vi "数据索引起始时间填补空白.vi"(8 "error in (no error)":errorcluster caption="错误输入（无错误）") -> (0 "error out":errorcluster caption="错误输出")   [LabVIEW 2016, in "数据传输系统.lvlib"]
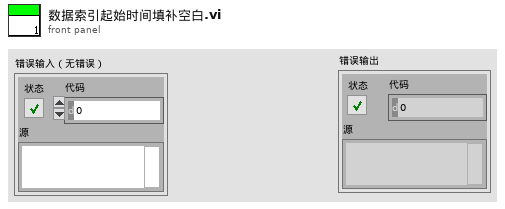
[diagram p1: front panel]
types:
  T1 = typedef "LVDateTimeRec.ctl" = cluster{"秒数的小数部分":dbl, "秒":i32, "分":i32, "时":i32, "日":i32, "月":i32, "年":i32, "天数（周）":i32, "天数（年）":i32, "DST":i32}
  T2 = cluster{"氨氮仪器参数索引起始时间":string, "总磷仪器参数索引起始时间":string, "总氮仪器参数索引起始时间":string, "CODMn仪器参数索引起始时间":string, "CODCr仪器参数索引起始时间":string, "DO仪器参数索引起始时间":string, "PH仪器参数索引起始时间":string, "比电导率仪器参数索引起始时间":string, "水温仪器参数索引起始时间":string, "浊度仪器参数索引起始时间":string, "叶绿素a仪器参数索引起始时间":string, "藻密度仪器参数索引起始时间":string, "ORP仪器参数索引起始时间":string}
  T3 = cluster{"氨氮标样核查索引起始时间":string, "总磷标样核查索引起始时间":string, "总氮标样核查索引起始时间":string, "CODMn标样核查索引起始时间":string, "CODCr标样核查索引起始时间":string, "DO标样核查索引起始时间":string, "PH标样核查索引起始时间":string, "比电导率标样核查索引起始时间":string, "水温标样核查索引起始时间":string, "浊度标样核查索引起始时间":string, "叶绿素a标样核查索引起始时间":string, "藻密度标样核查索引起始时间":string, "亚硝酸盐标样核查索引起始时间":string, "硫化物标样核查索引起始时间":string, "ORP标样核查索引起始时间":string}
  T4 = cluster{"氨氮跨度核查索引起始时间":string, "总磷跨度核查索引起始时间":string, "总氮跨度核查索引起始时间":string, "CODMn跨度核查索引起始时间":string, "CODCr跨度核查索引起始时间":string, "亚硝酸盐跨度核查索引起始时间":string, "硫化物跨度核查索引起始时间":string, "ORP跨度核查索引起始时间":string}
  T5 = cluster{"氨氮报警信息索引起始时间":string, "总磷报警信息索引起始时间":string, "总氮报警信息索引起始时间":string, "CODMn报警信息索引起始时间":string, "CODCr报警信息索引起始时间":string, "DO报警信息索引起始时间":string, "PH报警信息索引起始时间":string, "比电导率报警信息索引起始时间":string, "水温报警信息索引起始时间":string, "浊度报警信息索引起始时间":string, "叶绿素报警信息索引起始时间":string, "系统报警信息索引起始时间":string}
  T6 = cluster{"氨氮集成干预索引起始时间":string, "总磷集成干预索引起始时间":string, "总氮集成干预索引起始时间":string, "CODMn集成干预索引起始时间":string, "CODCr集成干预索引起始时间":string, "DO集成干预索引起始时间":string, "PH集成干预索引起始时间":string, "比电导率集成干预索引起始时间":string, "水温集成干预索引起始时间":string, "浊度集成干预索引起始时间":string, "叶绿素a集成干预索引起始时间":string, "藻密度集成干预索引起始时间":string, "亚硝酸盐集成干预索引起始时间":string, "硫化物集成干预索引起始时间":string, "ORP集成干预索引起始时间":string}
  T7 = cluster{"氨氮仪器日志索引起始时间":string, "总磷仪器日志索引起始时间":string, "总氮仪器日志索引起始时间":string, "CODMn仪器日志索引起始时间":string, "CODCr仪器日志索引起始时间":string, "系统仪器日志索引起始时间":string}
  T8 = cluster{"氨氮零点核查索引起始时间":string, "总磷零点核查索引起始时间":string, "总氮零点核查索引起始时间":string, "CODMn零点核查索引起始时间":string, "CODCr零点核查索引起始时间":string, "亚硝酸盐零点核查索引起始时间":string, "硫化物零点核查索引起始时间":string, "ORP零点核查索引起始时间":string}
  T9 = cluster{"氨氮平行样索引起始时间":string, "总磷平行样索引起始时间":string, "总氮平行样索引起始时间":string, "CODMn平行样索引起始时间":string, "CODCr平行样索引起始时间":string}
  T10 = cluster{"[0]":string, "[1]":string, "[2]":string, "[3]":string, "[4]":string, "[5]":string, "[6]":string, "[7]":string, "[8]":string, "[9]":string, "[10]":string, "[11]":string, "[12]":string}
  T11 = cluster{"[0]":string, "[1]":string, "[2]":string, "[3]":string, "[4]":string, "[5]":string, "[6]":string, "[7]":string, "[8]":string, "[9]":string, "[10]":string, "[11]":string, "[12]":string, "[13]":string, "[14]":string}
  T12 = cluster{"[0]":string, "[1]":string, "[2]":string, "[3]":string, "[4]":string}
  T13 = cluster{"[0]":string, "[1]":string, "[2]":string, "[3]":string, "[4]":string, "[5]":string, "[6]":string, "[7]":string}
  T14 = cluster{"[0]":string, "[1]":string, "[2]":string, "[3]":string, "[4]":string, "[5]":string, "[6]":string, "[7]":string, "[8]":string, "[9]":string, "[10]":string, "[11]":string}
  T15 = cluster{"[0]":string, "[1]":string, "[2]":string, "[3]":string, "[4]":string, "[5]":string}
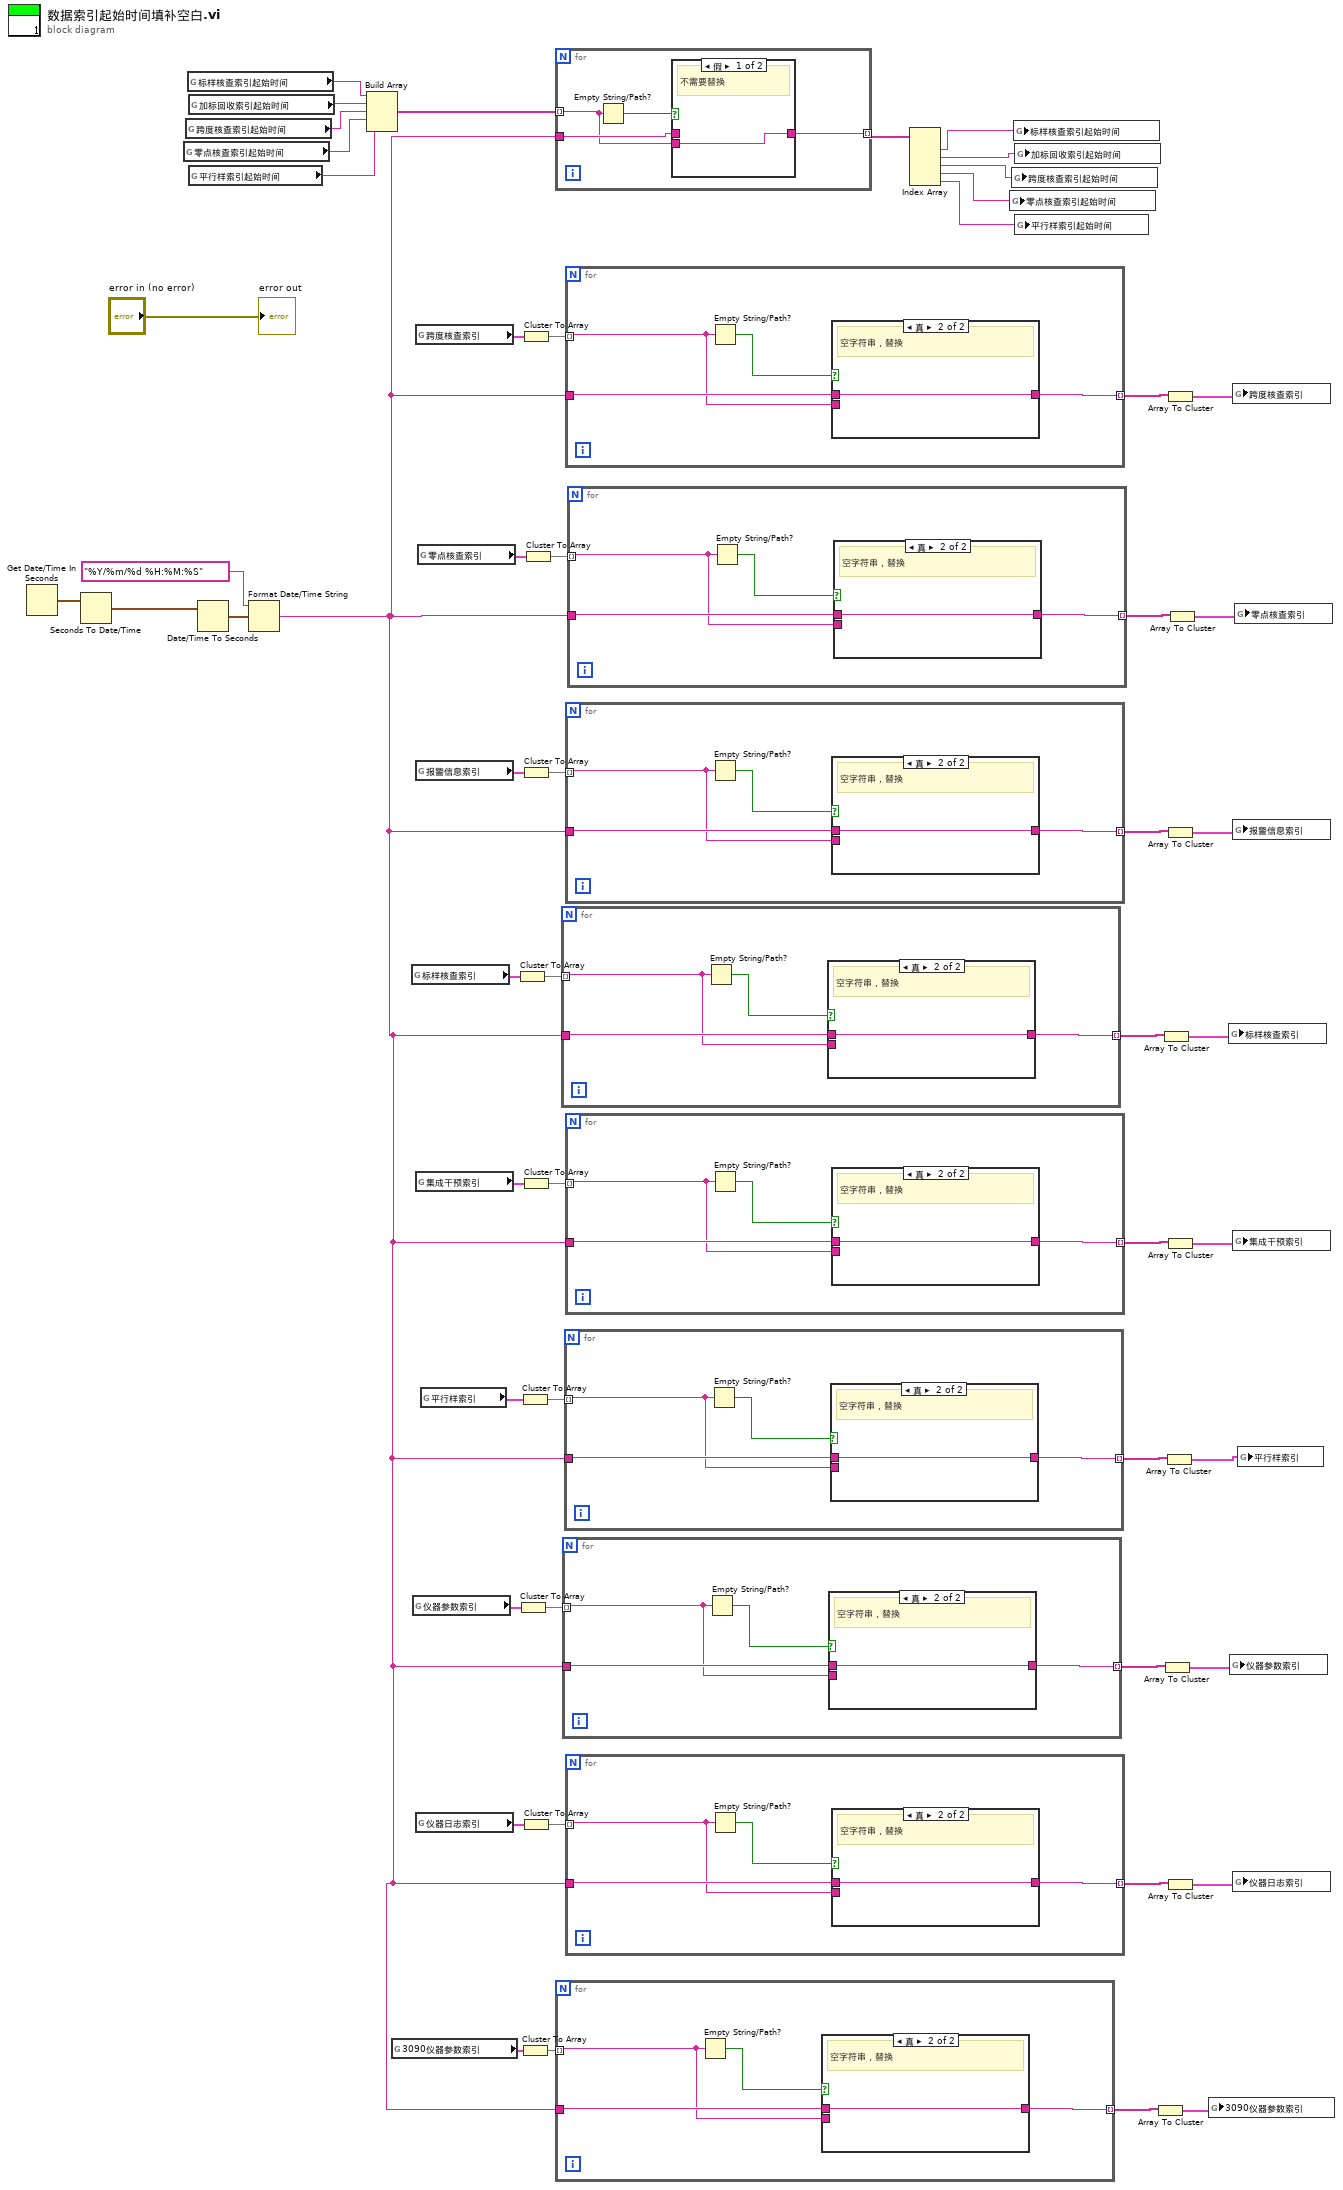
[diagram p0: block diagram]
diagram:
  n1 = Get Date/Time In Seconds() -> (seconds since 1Jan1904=w54:timestamp)
  n2 = Seconds To Date/Time(time stamp (now)=w54) -> (date time rec=w52:T1)  [unwired: 1 in]
  n3 = global read "全局 时间2.vi" "零点核查索引起始时间"() -> (w13:string)
  n4 = global read "全局 时间2.vi" "跨度核查索引起始时间"() -> (w15:string)
  n5 = global read "全局 时间2.vi" "标样核查索引起始时间"() -> (w17:string)
  n6 = global read "全局 时间2.vi" "加标回收索引起始时间"() -> (w16:string)
  n7 = global read "全局 时间2.vi" "平行样索引起始时间"() -> (w14:string)
  n8 = Date/Time To Seconds(2:w52) -> (0:w51:timestamp)  [unwired: 1 in]
  n9 = Format Date/Time String(time format string (%c)="%Y/%m/%d %H:%M:%S" ("时间格式字符串(%c)"), seconds (now)=w51) -> (date/time string=w1:string)  [unwired: 1 in]
  n10 = Build Array(w17, w16, w15, w13, w14) -> (w12:string[])
  n11 = global read "全局 时间2.vi" "3090仪器参数索引"() -> (w5:T2)
  n12 = global read "全局 时间2.vi" "标样核查索引"() -> (w42:T3)
  n13 = global read "全局 时间2.vi" "仪器参数索引"() -> (w23:T2)
  n14 = global read "全局 时间2.vi" "跨度核查索引"() -> (w31:T4)
  n15 = global read "全局 时间2.vi" "报警信息索引"() -> (w43:T5)
  n16 = global read "全局 时间2.vi" "集成干预索引"() -> (w35:T6)
  n17 = global read "全局 时间2.vi" "仪器日志索引"() -> (w22:T7)
  n18 = global read "全局 时间2.vi" "零点核查索引"() -> (w50:T8)
  n19 = global read "全局 时间2.vi" "平行样索引"() -> (w30:T9)
  n20 = Cluster To Array(cluster=w42) -> (array=w41:string[])
  n21 = Cluster To Array(cluster=w23) -> (array=w24:string[])
  n22 = Cluster To Array(cluster=w30) -> (array=w29:string[])
  n23 = Cluster To Array(cluster=w5) -> (array=w4:string[])
  n24 = Cluster To Array(cluster=w31) -> (array=w32:string[])
  n25 = Cluster To Array(cluster=w43) -> (array=w44:string[])
  n26 = Cluster To Array(cluster=w35) -> (array=w36:string[])
  n27 = Cluster To Array(cluster=w22) -> (array=w21:string[])
  n28 = Cluster To Array(cluster=w50) -> (array=w49:string[])
  n29 = for {
    tunnel: w12 -> [w56] mode=indexing
    tunnel: w1 -> [w57]
    tunnel: [w55] -> w11 mode=indexing
    n30 = Empty String/Path?(string/path=w56) -> (empty?=w58:bool)
    n31 = case shown="假" w58 {
      tunnel: w57 -> [_ w60]
      tunnel: [w59 w60] -> w55
      tunnel: w56 -> [w59 _]
      frame False {
        # "不需要替换"
      }
      frame True {
        # "空字符串，替换"
      }
    }
  }
  n32 = for {
    tunnel: w4 -> [w61] mode=indexing
    tunnel: w1 -> [w63]
    tunnel: [w62] -> w3 mode=indexing
    n33 = Empty String/Path?(string/path=w61) -> (empty?=w64:bool)
    n34 = case shown="真" w64 {
      tunnel: w63 -> [_ w66]
      tunnel: [w65 w66] -> w62
      tunnel: w61 -> [w65 _]
      frame False {
        # "不需要替换"
      }
      frame True {
        # "空字符串，替换"
      }
    }
  }
  n35 = for {
    tunnel: w41 -> [w67] mode=indexing
    tunnel: w1 -> [w69]
    tunnel: [w68] -> w40 mode=indexing
    n36 = Empty String/Path?(string/path=w67) -> (empty?=w70:bool)
    n37 = case shown="真" w70 {
      tunnel: w69 -> [_ w72]
      tunnel: [w71 w72] -> w68
      tunnel: w67 -> [w71 _]
      frame False {
        # "不需要替换"
      }
      frame True {
        # "空字符串，替换"
      }
    }
  }
  n38 = for {
    tunnel: w24 -> [w73] mode=indexing
    tunnel: w1 -> [w75]
    tunnel: [w74] -> w25 mode=indexing
    n39 = Empty String/Path?(string/path=w73) -> (empty?=w76:bool)
    n40 = case shown="真" w76 {
      tunnel: w75 -> [_ w78]
      tunnel: [w77 w78] -> w74
      tunnel: w73 -> [w77 _]
      frame False {
        # "不需要替换"
      }
      frame True {
        # "空字符串，替换"
      }
    }
  }
  n41 = for {
    tunnel: w29 -> [w79] mode=indexing
    tunnel: w1 -> [w81]
    tunnel: [w80] -> w28 mode=indexing
    n42 = Empty String/Path?(string/path=w79) -> (empty?=w82:bool)
    n43 = case shown="真" w82 {
      tunnel: w81 -> [_ w84]
      tunnel: [w83 w84] -> w80
      tunnel: w79 -> [w83 _]
      frame False {
        # "不需要替换"
      }
      frame True {
        # "空字符串，替换"
      }
    }
  }
  n44 = for {
    tunnel: w32 -> [w85] mode=indexing
    tunnel: w1 -> [w87]
    tunnel: [w86] -> w33 mode=indexing
    n45 = Empty String/Path?(string/path=w85) -> (empty?=w88:bool)
    n46 = case shown="真" w88 {
      tunnel: w87 -> [_ w90]
      tunnel: [w89 w90] -> w86
      tunnel: w85 -> [w89 _]
      frame False {
        # "不需要替换"
      }
      frame True {
        # "空字符串，替换"
      }
    }
  }
  n47 = for {
    tunnel: w44 -> [w91] mode=indexing
    tunnel: w1 -> [w93]
    tunnel: [w92] -> w45 mode=indexing
    n48 = Empty String/Path?(string/path=w91) -> (empty?=w94:bool)
    n49 = case shown="真" w94 {
      tunnel: w93 -> [_ w96]
      tunnel: [w95 w96] -> w92
      tunnel: w91 -> [w95 _]
      frame False {
        # "不需要替换"
      }
      frame True {
        # "空字符串，替换"
      }
    }
  }
  n50 = for {
    tunnel: w36 -> [w97] mode=indexing
    tunnel: w1 -> [w99]
    tunnel: [w98] -> w37 mode=indexing
    n51 = Empty String/Path?(string/path=w97) -> (empty?=w100:bool)
    n52 = case shown="真" w100 {
      tunnel: w99 -> [_ w102]
      tunnel: [w101 w102] -> w98
      tunnel: w97 -> [w101 _]
      frame False {
        # "不需要替换"
      }
      frame True {
        # "空字符串，替换"
      }
    }
  }
  n53 = for {
    tunnel: w21 -> [w103] mode=indexing
    tunnel: w1 -> [w105]
    tunnel: [w104] -> w20 mode=indexing
    n54 = Empty String/Path?(string/path=w103) -> (empty?=w106:bool)
    n55 = case shown="真" w106 {
      tunnel: w105 -> [_ w108]
      tunnel: [w107 w108] -> w104
      tunnel: w103 -> [w107 _]
      frame False {
        # "不需要替换"
      }
      frame True {
        # "空字符串，替换"
      }
    }
  }
  n56 = for {
    tunnel: w49 -> [w109] mode=indexing
    tunnel: w1 -> [w111]
    tunnel: [w110] -> w48 mode=indexing
    n57 = Empty String/Path?(string/path=w109) -> (empty?=w112:bool)
    n58 = case shown="真" w112 {
      tunnel: w111 -> [_ w114]
      tunnel: [w113 w114] -> w110
      tunnel: w109 -> [w113 _]
      frame False {
        # "不需要替换"
      }
      frame True {
        # "空字符串，替换"
      }
    }
  }
  n59 = Index Array(array=w11) -> (element #1=w10:string, element #2=w9:string, element #3=w8:string, element #4=w6:string, element #5=w7:string)  [unwired: 5 in]
  n60 = global write "全局 时间2.vi" "零点核查索引起始时间"(w6) -> ()
  n61 = global write "全局 时间2.vi" "跨度核查索引起始时间"(w8) -> ()
  n62 = global write "全局 时间2.vi" "标样核查索引起始时间"(w10) -> ()
  n63 = global write "全局 时间2.vi" "加标回收索引起始时间"(w9) -> ()
  n64 = global write "全局 时间2.vi" "平行样索引起始时间"(w7) -> ()
  n65 = Array To Cluster(array=w3) -> (cluster=w2:T10)
  n66 = Array To Cluster(array=w40) -> (cluster=w39:T11)
  n67 = Array To Cluster(array=w25) -> (cluster=w26:T10)
  n68 = Array To Cluster(array=w28) -> (cluster=w27:T12)
  n69 = Array To Cluster(array=w33) -> (cluster=w34:T13)
  n70 = Array To Cluster(array=w45) -> (cluster=w46:T14)
  n71 = Array To Cluster(array=w37) -> (cluster=w38:T11)
  n72 = Array To Cluster(array=w20) -> (cluster=w19:T15)
  n73 = Array To Cluster(array=w48) -> (cluster=w47:T13)
  n74 = global write "全局 时间2.vi" "3090仪器参数索引"(w2) -> ()
  n75 = global write "全局 时间2.vi" "标样核查索引"(w39) -> ()
  n76 = global write "全局 时间2.vi" "仪器参数索引"(w26) -> ()
  n77 = global write "全局 时间2.vi" "跨度核查索引"(w34) -> ()
  n78 = global write "全局 时间2.vi" "报警信息索引"(w46) -> ()
  n79 = global write "全局 时间2.vi" "集成干预索引"(w38) -> ()
  n80 = global write "全局 时间2.vi" "仪器日志索引"(w19) -> ()
  n81 = global write "全局 时间2.vi" "零点核查索引"(w47) -> ()
  n82 = global write "全局 时间2.vi" "平行样索引"(w27) -> ()
  "error out" <- "error in (no error)"
